vi "test4-Message_Queue.vi"(8 "error in (no error)":errorcluster, 11 "TestCase in":refnum<class "testcase-CSMGlobalLog.lvclass">) -> (0 "error out":errorcluster, 3 "TestCase out":refnum<class "testcase-CSMGlobalLog.lvclass">)   [LabVIEW 2017, in "testcase-CSMGlobalLog.lvclass"]
uses:
  testcase-CSMGlobalLog.lvclass
  testcase-CSMGlobalLog.lvclass/testcase-CSMGlobalLog.ctl
  src/user.lib/_NEVSTOP/Communicable State Machine(CSM)/Utility/Periodic String Filter Setting.ctl
  <vilib>/addons/_JKI Toolkits/VI Tester/TestCase.llb/TestCase.lvclass
  src/user.lib/_NEVSTOP/Communicable State Machine(CSM)/Communicable State Machine.lvlib
  C:/Program Files (x86)/National Instruments/LabVIEW 2017/vi.lib/addons/_JKI Toolkits/VI Tester/TestCase.llb/TestCase.lvclass
panel:
  out "error out 3":errorcluster
  out "LoopCount":i32
  out "String Cache Total":string
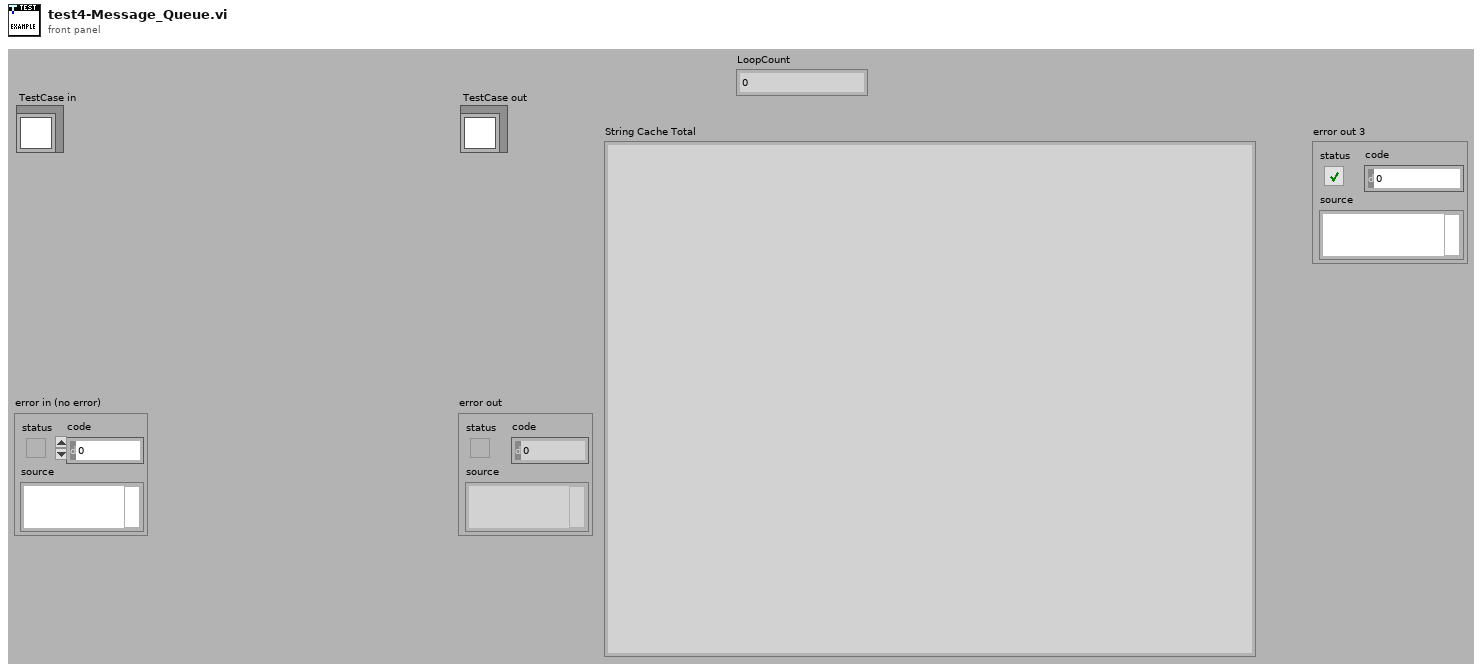
[diagram p1: front panel]
types:
  T1 = typedef "Communicable State Machine.lvlib/Periodic String Filter Setting.ctl" = cluster{"threashold(#/s)":dbl, "Check Peroid(s)":dbl}
  T2 = typedef "Communicable State Machine.lvlib/_CSM_GlobalLog_MSG.ctl" = cluster{"Name (\"\" to Use UUID)":string, "Current State":string, "Arguments":string, "Source Message":T3, "Source Module":string, "Complete(T)/Start(F)":bool, "LogType":T4, "Time Stamp":timestamp}
  T3 = typedef "Communicable State Machine.lvlib/_CSM_Response Source Message.ctl" = cluster{"‘State":string, "’Arguments":string, "’Error":errorcluster}
  T4 = typedef "Communicable State Machine.lvlib/_CSM_GlobalLog_MSG_TYPE.ctl" = enum16{"User Log", "State Change", "Status", "Interrupt", "Register", "Unregister", "Error Log", "Module Created", "Module Destroyed"}
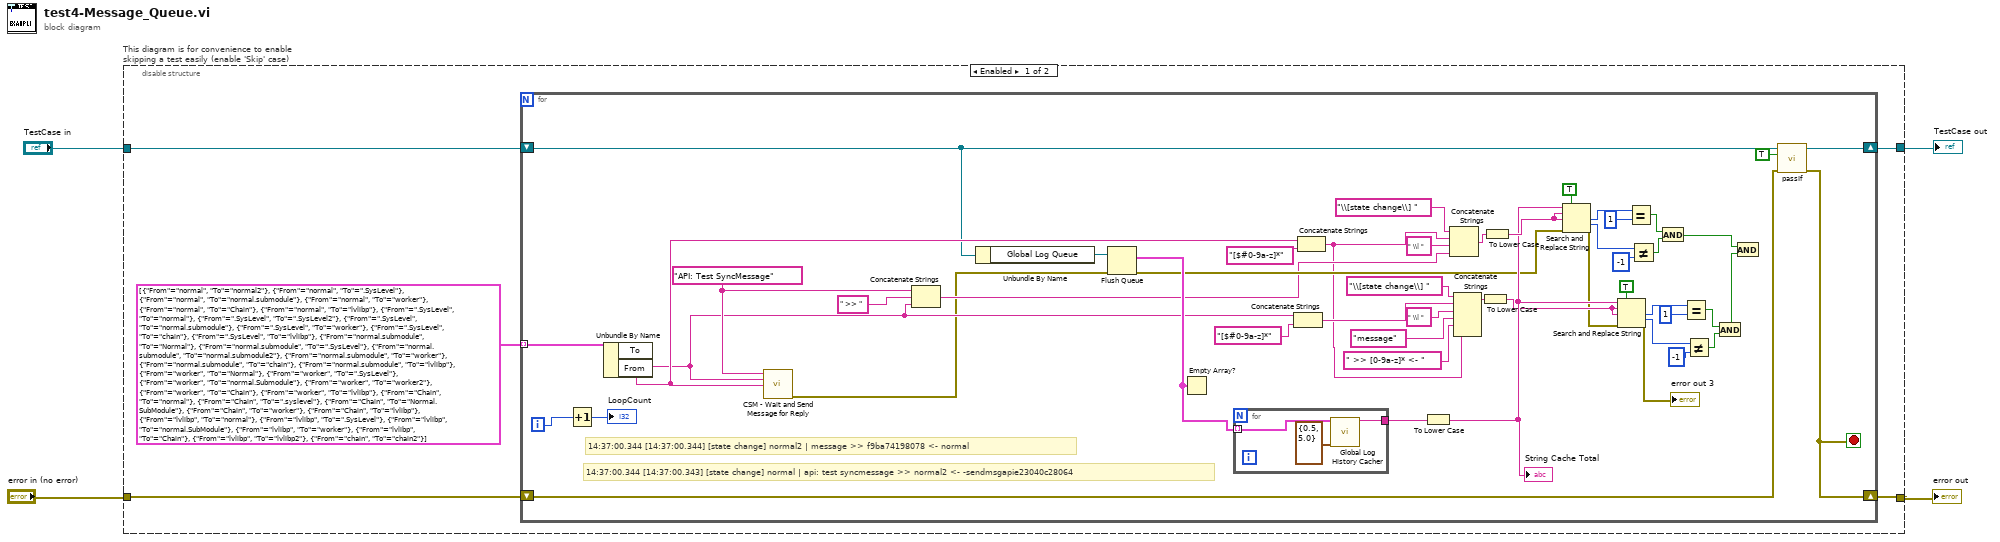
[diagram p0: block diagram]
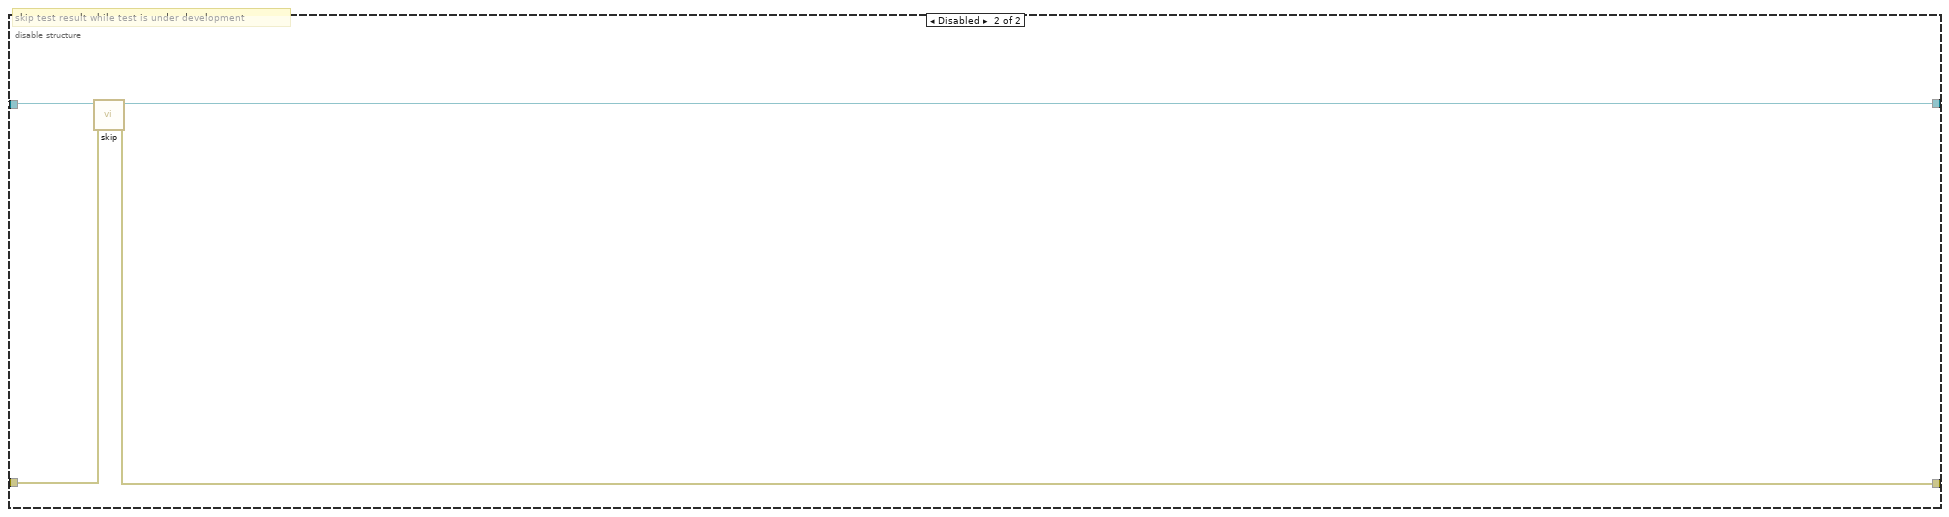
[diagram p2: hidden frame]
diagram:
  n1 = disable-structure "This diagram is for convenience to enable skipping a test easily (enable 'Skip' case)" shown="Enabled" {
    disable-tunnel: "TestCase in" -> [w5 w67]
    disable-tunnel: [w8 w65] -> w1
    disable-tunnel: [w9 w66] -> w3
    disable-tunnel: "error in (no error)" -> [w7 w64]
    frame Enabled {
      n2 = for {
        tunnel: cluster{"From":string, "To":string}[] [{"From"="normal", "To"="normal2"}, {"From"="normal", "To"=".SysLevel"}, {"From"="normal", "To"="normal.submodule"}, {"From"="normal", "To"="worker"}, {"From"="normal", "To"="Chain"}, {"From"="normal", "To"="lvlibp"}, {"From"=".SysLevel", "To"="normal"}, {"From"=".SysLevel", "To"=".SysLevel2"}, {"From"=".SysLevel", "To"="normal.submodule"}, {"From"=".SysLevel", "To"="worker"}, {"From"=".SysLevel", "To"="chain"}, {"From"=".SysLevel", "To"="lvlibp"}, {"From"="normal.submodule", "To"="Normal"}, {"From"="normal.submodule", "To"=".SysLevel"}, {"From"="normal.submodule", "To"="normal.submodule2"}, {"From"="normal.submodule", "To"="worker"}, {"From"="normal.submodule", "To"="chain"}, {"From"="normal.submodule", "To"="lvlibp"}, {"From"="worker", "To"="Normal"}, {"From"="worker", "To"=".SysLevel"}, {"From"="worker", "To"="normal.Submodule"}, {"From"="worker", "To"="worker2"}, {"From"="worker", "To"="Chain"}, {"From"="worker", "To"="lvlibp"}, {"From"="Chain", "To"="normal"}, {"From"="Chain", "To"=".syslevel"}, {"From"="Chain", "To"="Normal.SubModule"}, {"From"="Chain", "To"="worker"}, {"From"="Chain", "To"="lvlibp"}, {"From"="lvlibp", "To"="normal"}, {"From"="lvlibp", "To"=".SysLevel"}, {"From"="lvlibp", "To"="normal.SubModule"}, {"From"="lvlibp", "To"="worker"}, {"From"="lvlibp", "To"="Chain"}, {"From"="lvlibp", "To"="lvlibp2"}, {"From"="chain", "To"="chain2"}] -> [w32] mode=indexing
        shift-right: [w11] -> w9
        shift-left: w7 -> [w58]
        shift-right: [w60] -> w8
        shift-left: w5 -> [w13]
        i -> [w57]
        stop <- w11 stop-if-true
        w22 = "API: Test SyncMessage" ("State")
        # "14:37:00.344 [14:37:00.344] [state change] normal2 | message >> f9ba74198078 <- normal"
        # "14:37:00.344 [14:37:00.343] [state change] normal | api: test syncmessage >> normal2 <- -sendmsgapie23040c28064"
        n3 = Increment(x=w57) -> (x+1=→"LoopCount":i32)
        n4 = Unbundle By Name(w32) -> ("To"=w18:string, "From"=w23:string)
        n5 = call "CSM - Wait and Send Message for Reply.vi"("State"=w22, "Arguments (\"\")"=w18, "Target Module"=w23) -> ("error out"=w10:errorcluster)  [unwired: 10 in, 2 out]
        n6 = Concatenate Strings(w22, " >> " ("string"), w18) -> (w21:string)
        n7 = Unbundle By Name(w13) -> ("Global Log Queue"=w59:refnum<queue>)
        n8 = Flush Queue(queue=w59, error in (no error)=w10) -> (remaining elements=w55:T2[], error out=w37:errorcluster)  [unwired: 1 out]
        n9 = Empty Array?(array=w55) -> ()  [unwired: 1 out]
        n10 = for {
          tunnel: w55 -> [w63] mode=indexing
          tunnel: [w62] -> w12
          n11 = call "Global Log History Cacher.vi"("Global Log Data"=w63, "Settings"=T1 {"threashold(#/s)"=0.5, "Check Peroid(s)"=5.0}) -> ("String Cache"=w62:string)  [unwired: 13 in]
        }
        n12 = Concatenate Strings(w18, "[$#0-9a-z]*" ("string")) -> (w17:string)
        n13 = Concatenate Strings(w23, "[$#0-9a-z]*" ("string")) -> (w14:string)
        n14 = To Lower Case(string=w12) -> (all lower case string=w41:string)
        "String Cache Total" <- w41
        n15 = Concatenate Strings("\\[state change\\] " ("regular expression"), w14, " \\| " ("string"), w21) -> (w27:string)
        n16 = Concatenate Strings("\\[state change\\] " ("regular expression"), w17, " \\| " ("string"), "message" ("string"), " >> [0-9a-z]* <- ", w14) -> (w29:string)
        n17 = To Lower Case(string=w29) -> (all lower case string=w40:string)
        n18 = To Lower Case(string=w27) -> (all lower case string=w53:string)
        n19 = Search and Replace String(replace all?=TRUE ("replace all? (F)"), input string=w41, search string=w53, replace string=w53, error in=w37) -> (number of replacements=w52:i32, offset past replacement=w51:i32, error out=w39:errorcluster)  [unwired: 3 in, 1 out]
        n20 = Search and Replace String(replace all?=TRUE ("replace all? (F)"), input string=w41, search string=w40, replace string=w40, error in=w39) -> (number of replacements=w43:i32, offset past replacement=w44:i32, error out=→"error out 3":errorcluster)  [unwired: 3 in, 1 out]
        n21 = Equal?(x=w52, y=1) -> (x = y?=w49:bool)
        n22 = Not Equal?(x=w51, y=-1) -> (x != y?=w48:bool)
        n23 = And(x=w49, y=w48) -> (x .and. y?=w33:bool)
        n24 = Equal?(x=w43, y=1) -> (x = y?=w46:bool)
        n25 = Not Equal?(x=w44, y=-1) -> (x != y?=w47:bool)
        n26 = And(x=w46, y=w47) -> (x .and. y?=w38:bool)
        n27 = And(x=w33, y=w38) -> ()  [unwired: 1 out]
        n28 = call-dynamic "passIf.vi"("error in (no error)"=w58, "pass"=TRUE, "TestCase in"=w13) -> ("error out"=w11:errorcluster, "TestCase out"=w60:refnum<class "testcase-CSMGlobalLog.lvclass">)  [unwired: 7 in]
      }
    }
    frame Disabled {
      # "skip test result while test is under development"
      n29 = call <vilib>:"skip.vi"("error in (no error)"=w64, "TestCase in"=w67) -> ("error out"=w66:errorcluster, "TestCase out"=w65:refnum<class "testcase-CSMGlobalLog.lvclass">)  [unwired: 8 in]
    }
  }
  "error out" <- w3
  "TestCase out" <- w1
